vi "Get 3.5 char times.vi"(11 "baud rate":u32) -> (3 "wait time (ms)":u32, 5 "default wait (ms)":u32)   [LabVIEW 2017, in "SubVIs.lvlib" / "Serial Shared Components.lvlib"]
uses:
  <vilib>/Modbus/subvis/Protocol/Serial/Serial Shared Components/Serial Shared Components.lvlib
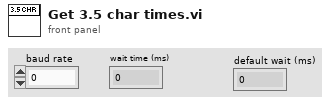
[diagram p1: front panel]
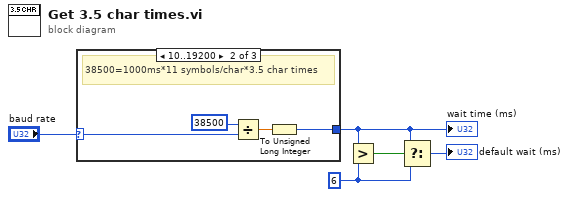
[diagram p0: block diagram]
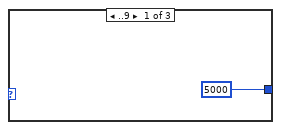
[diagram p2: hidden frame]
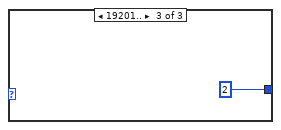
[diagram p3: hidden frame]
diagram:
  w2 = u32 6 ("y")
  n1 = case shown="10..19200" "baud rate" {
    selector: "baud rate" -> [_ w9 _]
    tunnel: [u32 5000 w7 u32 2] -> w3
    frame ..9 {
    }
    frame 10..19200 {
      # "38500=1000ms*11 symbols/char*3.5 char times"
      n2 = Divide(x=u32 38500 ("y"), y=w9) -> (x/y=w10:dbl)
      n3 = To Unsigned Long Integer(number=w10) -> (unsigned 32bit integer=w7:u32)
    }
    frame 19201.. {
    }
  }
  "wait time (ms)" <- w3
  n4 = Greater?(x=w3, y=w2) -> (0:w4:bool)
  n5 = Select(t=w3, s=w4, f=w2) -> (s? t:f=→"default wait (ms)":u32)
